vi "Clear Status.vi"(8 "error":errorcluster, 11 "VISA":refnum<visa-resource-name>) -> (0 "error out":errorcluster, 3 "VISA out":refnum<visa-resource-name>)   [LabVIEW 2025, in "TDK-Lambda GEN LAN Series.lvlib"]
doc: "Sends \"*CLS\" to clear the status registers including:\n- System Error queue\n- Output queue\n- Standard Event register\n- Operational Event registers\n- Conditional Event registers\n- Status Byte"
uses:
  <userlib>/TDK-Lambda GEN LAN Series/TDK-Lambda GEN LAN Series.lvlib
panel:
  in  "Slave Address":i32=-1 min=-1 max=30 step=1
  # "TDK-Lambda Genesys \n LAN\n  DC Power Supplies"
  # "Clear Status"
  # "(c) 2019 TDK-Lambda.  ALL RIGHTS RESERVED."
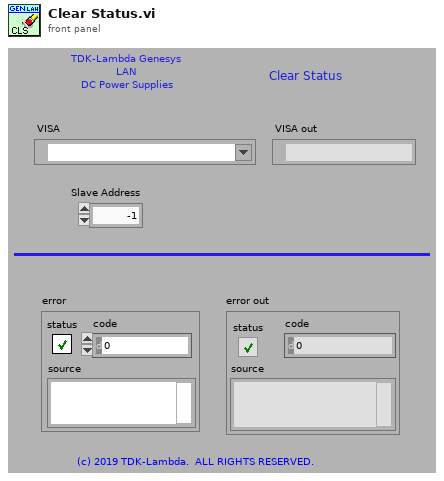
[diagram p1: front panel]
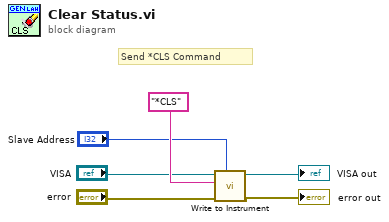
[diagram p0: block diagram]
diagram:
  # "Send *CLS Command"
  n1 = call <userlib>:"Write to Instrument.vi"("Slave Address"="Slave Address", "error"="error", "Command"="*CLS", "VISA"="VISA") -> ("error out"=→"error out":errorcluster, "VISA out"=→"VISA out":refnum<visa-resource-name>)  [unwired: 6 in]
